vi "Read Scan file parsed_.vi"(8 "error in (no error)":errorcluster, 11 "HC-Main in":refnum<class "HC-Main.lvclass">) -> (0 "error out":errorcluster, 2 "Scan file parsed?":bool, 3 "HC-Main out":refnum<class "HC-Main.lvclass">)   [LabVIEW 2013, in "HardwareCharacterization.lvlib" / "HC-Main.lvclass"]
uses:
  HC-Main.lvclass
  HC-Main.lvclass/HC-Main.ctl
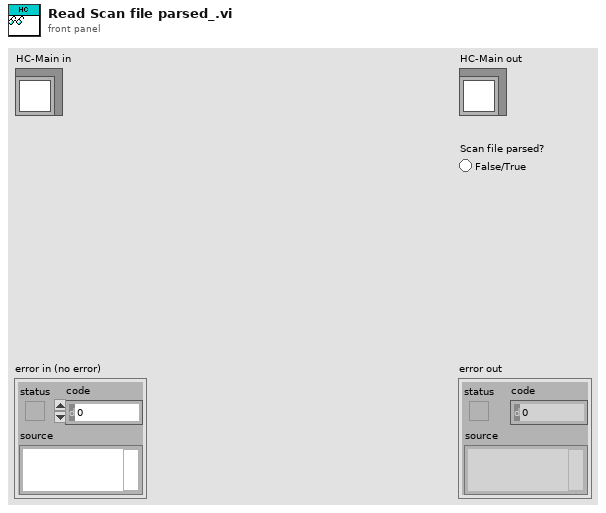
[diagram p1: front panel]
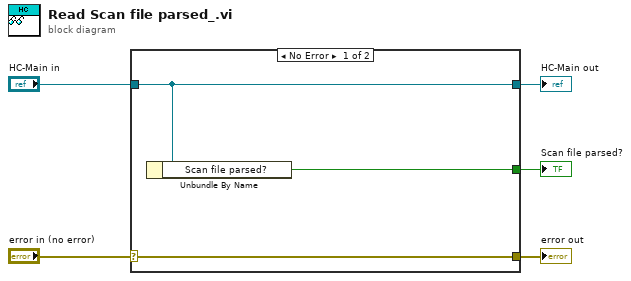
[diagram p0: block diagram]
diagram:
  n1 = case shown="No Error" "error in (no error)" {
    selector: "error in (no error)" -> [w8 w9]
    tunnel: [w8 w9] -> w4
    tunnel: [w7 w10] -> w2
    tunnel: "HC-Main in" -> [w7 w10]
    tunnel: [w6 _] -> w1
    frame No Error {
      n2 = Unbundle By Name(w7) -> ("Scan file parsed?"=w6:bool)
    }
    frame Error {
    }
  }
  "error out" <- w4
  "HC-Main out" <- w2
  "Scan file parsed?" <- w1
